vi "Read transfer info.vi"(8 "error in (no error)":errorcluster, 11 "DSFTransfer in":refnum<class "DSFTransfer.lvclass">) -> (0 "error out":errorcluster, 2 "transfer info":T1, 3 "DSFTransfer out":refnum<class "DSFTransfer.lvclass">)   [LabVIEW 2017, in "DSFTransfer.lvclass"]
uses:
  DSFTransfer.lvclass
  Controls/dsf transfer.ctl
  DSFTransfer.lvclass/DSFTransfer.ctl
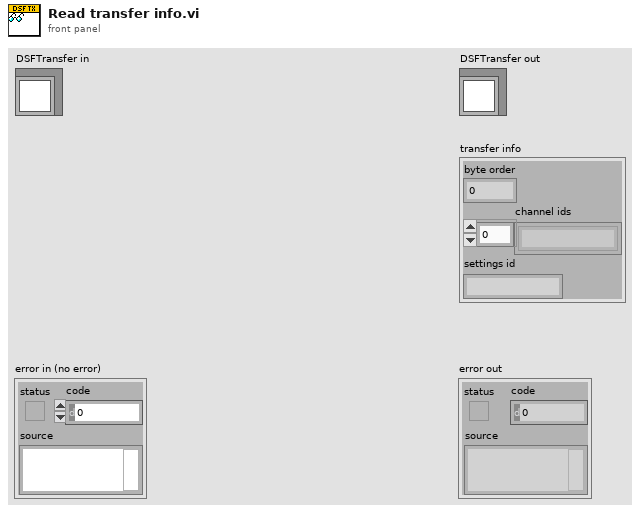
[diagram p1: front panel]
types:
  T1 = typedef "dsf transfer.ctl" = cluster{"byte order":i32, "channel ids":string[], "settings id":string}
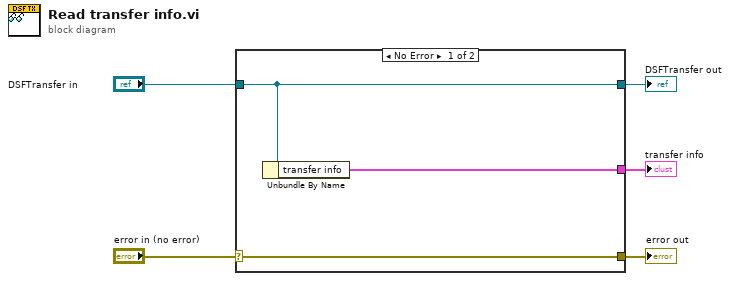
[diagram p0: block diagram]
diagram:
  n1 = case shown="No Error" "error in (no error)" {
    selector: "error in (no error)" -> [w8 w9]
    tunnel: [w8 w9] -> w4
    tunnel: [w7 w10] -> w2
    tunnel: "DSFTransfer in" -> [w7 w10]
    tunnel: [w6 _] -> w1
    frame No Error {
      n2 = Unbundle By Name(w7) -> ("transfer info"=w6:T1)
    }
    frame Error {
    }
  }
  "error out" <- w4
  "DSFTransfer out" <- w2
  "transfer info" <- w1
